vi "Next_Core.vi"(8 "error in (no error)":errorcluster, 10 "Query Result in":refnum<class "Query Result.lvclass">, 11 "SqlMapper in":refnum<class "SqlMapper.lvclass">) -> (0 "error out":errorcluster, 1 "Found":bool, 2 "Row as Variant":variant, 3 "SqlMapper out":refnum<class "SqlMapper.lvclass">)   [LabVIEW 2020, in "ORM.lvlib" / "Query Result.lvclass"]
uses:
  Query Result.lvclass
  SqlMapper/SqlMapper.lvclass
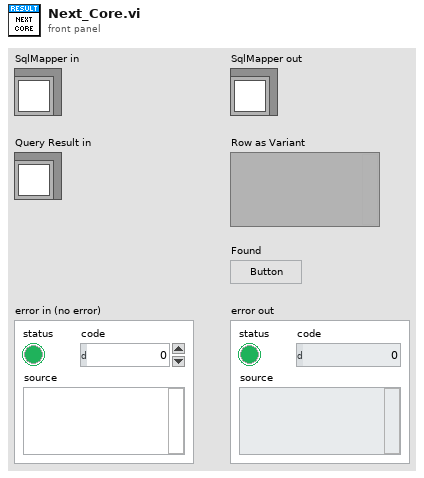
[diagram p1: front panel]
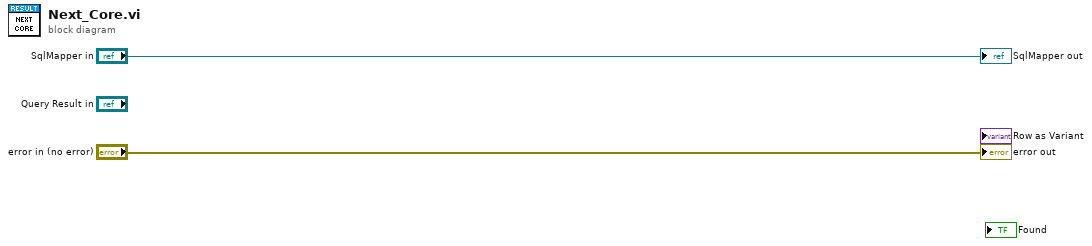
[diagram p0: block diagram]
diagram:
  "SqlMapper out" <- "SqlMapper in"
  "error out" <- "error in (no error)"
